vi "Array Max & Min PtByPt.vi"(0 "input data point":dbl format="%0.2f", 1 "sample length":i32=100, 2 "initialize":bool) -> (3 "error":i32, 4 "max index":i32, 5 "max value":dbl format="%0.2f", 6 "min index":i32, 7 "min value":dbl format="%0.2f")   [LabVIEW 2020, in "NI_PtbyPt.lvlib"]
doc: "Searches for the maximum and minimum values in the set of input data points specified by <B>sample length</B> where the region of interest is determined by the last <B>sample length</B> data. The indexes are between 0 and <B>sample length</B>."
uses:
  NI_PtbyPt.lvlib
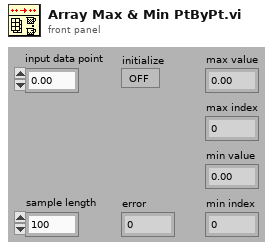
[diagram p1: front panel]
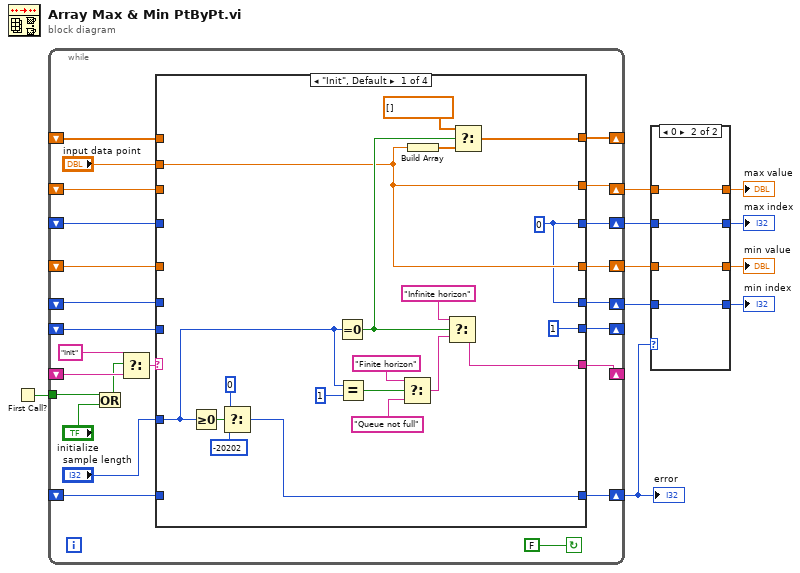
[diagram p0: block diagram]
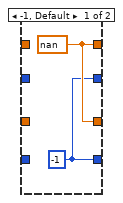
[diagram p2: hidden frame]
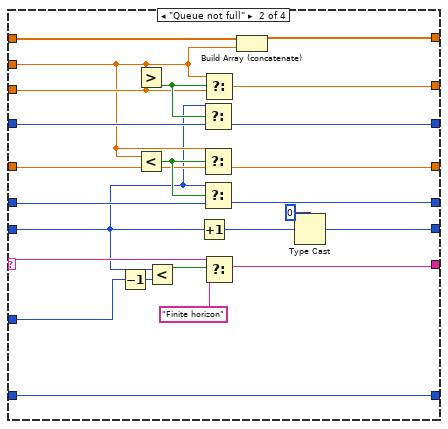
[diagram p3: hidden frame]
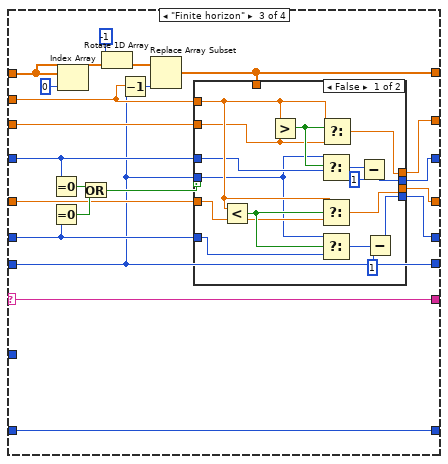
[diagram p4: hidden frame]
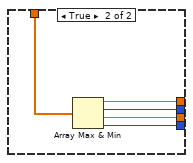
[diagram p5: hidden frame]
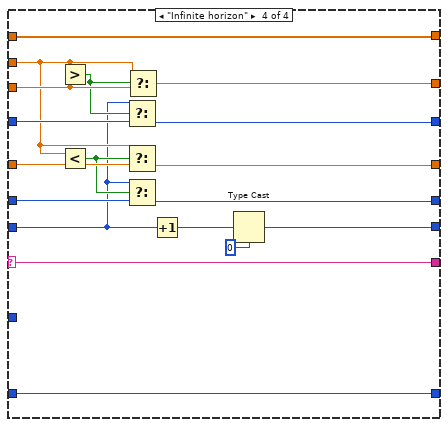
[diagram p6: hidden frame]
diagram:
  n1 = First Call?() -> (First Call?: T/F=w10:bool)
  n2 = while {
    tunnel: w10 -> [w15]
    shift-left: _ -> [w19]
    shift-right: [w22] -> w6
    shift-left: _ -> [w20]
    shift-right: [w21] -> w4
    shift-left: _ -> [w24]
    shift-right: [w23] -> w2
    shift-left: _ -> [w26]
    shift-right: [w25] -> _
    shift-left: _ -> [w28]
    shift-right: [w29] -> _
    shift-left: _ -> [w30]
    shift-right: [w31] -> w9
    shift-left: _ -> [w34]
    shift-right: [w27] -> _
    shift-right: [w12] -> w7
    shift-left: _ -> [w11]
    stop <- FALSE continue-if-true
    n3 = Or(x=w15, y="initialize") -> (x .or. y?=w13:bool)
    n4 = Select(t="Init", s=w13, f=w34) -> (s? t:f=w32:string)
    n5 = case shown="\"Init\", Default" w32 {
      selector: w32 -> [_ w70 w94 w137]
      tunnel: [w40 w60 w80 w125] -> w31
      tunnel: w30 -> [_ w61 w82 w126]
      tunnel: "input data point" -> [w41 w56 w86 w130]
      tunnel: [1 w74 w81 w122] -> w29
      tunnel: w28 -> [_ w55 w81 w124]
      tunnel: [w46 w68 w94 w137] -> w27
      tunnel: w26 -> [_ w77 w88 w136]
      tunnel: [w42 w76 w87 w136] -> w25
      tunnel: "sample length" -> [w38 w72 _ _]
      tunnel: w24 -> [_ w64 w85 w135]
      tunnel: [w41 w57 w90 w134] -> w23
      tunnel: [w41 w59 w89 w128] -> w22
      tunnel: [w40 w58 w79 w131] -> w21
      tunnel: w20 -> [_ w63 w84 w133]
      tunnel: w19 -> [_ w62 w83 w129]
      tunnel: [w35 w54 w78 w120] -> w12
      tunnel: w11 -> [_ w54 w78 w120]
      frame "Init", Default {
        w40 = 0
        n6 = Greater Or Equal To 0?(x=w38) -> (x >= 0?=w39:bool)
        n7 = Select(t=0, s=w39, f=-20202) -> (s? t:f=w35:i32)
        n8 = Equal To 0?(x=w38) -> (x = 0?=w45:bool)
        n9 = Equal?(x=w38, y=1) -> (x = y?=w50:bool)
        n10 = Select(t="Finite horizon", s=w50, f="Queue not full") -> (s? t:f=w48:string)
        n11 = Build Array(w41) -> (w44:dbl[])
        n12 = Select(t="Infinite horizon", s=w45, f=w48) -> (s? t:f=w46:string)
        n13 = Select(t=dbl[] [], s=w45, f=w44) -> (s? t:f=w42:dbl[])
      }
      frame "Queue not full" {
        n14 = Decrement(x=w72) -> (x-1=w67:i32)
        n15 = Greater?(x=w56, y=w64) -> (0:w66:bool)
        n16 = Less?(x=w56, y=w62) -> (x < y?=w65:bool)
        n17 = Less?(x=w55, y=w67) -> (x < y?=w71:bool)
        n18 = Increment(x=w55) -> (x+1=w75:i32)
        n19 = Select(t=w55, s=w66, f=w63) -> (s? t:f=w58:i32)
        n20 = Select(t=w56, s=w65, f=w62) -> (s? t:f=w59:dbl)
        n21 = Select(t=w55, s=w65, f=w61) -> (s? t:f=w60:i32)
        n22 = Select(t=w56, s=w66, f=w64) -> (s? t:f=w57:dbl)
        n23 = Select(t=w70, s=w71, f="Finite horizon") -> (s? t:f=w68:string)
        n24 = Build Array (concatenate)(w77, w56) -> (w76:dbl[])
        n25 = Type Cast(type=0, x=w75) -> (*(type *) &x=w74:i32)
      }
      frame "Finite horizon" {
        n26 = Equal To 0?(x=w84) -> (x = 0?=w93:bool)
        n27 = Equal To 0?(x=w82) -> (x = 0?=w92:bool)
        n28 = Index Array(array=w88, index=0 ("Index")) -> ()  [unwired: 1 out]
        n29 = Or(x=w93, y=w92) -> (x .or. y?=w91:bool)
        n30 = Rotate 1D Array(1:w88, 2:i16 -1 ("n")) -> (0:w96:dbl[])
        n31 = Decrement(x=w81) -> (x-1=w95:i32)
        n32 = Replace Array Subset(array=w96, new element=w86, index=w95) -> (w87:dbl[])
        n33 = case shown="False" w91 {
          tunnel: w87 -> [_ w119]
          tunnel: [w107 w118] -> w90
          tunnel: [w103 w117] -> w79
          tunnel: [w106 w116] -> w89
          tunnel: [w99 w115] -> w80
          tunnel: w86 -> [w112 _]
          tunnel: w85 -> [w111 _]
          tunnel: w84 -> [w108 _]
          tunnel: w83 -> [w110 _]
          tunnel: w82 -> [w109 _]
          tunnel: w81 -> [w105 _]
          frame False {
            n34 = Less?(x=w112, y=w110) -> (x < y?=w113:bool)
            n35 = Greater?(x=w112, y=w111) -> (0:w114:bool)
            n36 = Select(t=w105, s=w114, f=w108) -> (s? t:f=w104:i32)
            n37 = Select(t=w112, s=w113, f=w110) -> (s? t:f=w106:dbl)
            n38 = Select(t=w105, s=w113, f=w109) -> (s? t:f=w101:i32)
            n39 = Select(t=w112, s=w114, f=w111) -> (s? t:f=w107:dbl)
            n40 = Subtract(x=w104, y=1) -> (x-y=w103:i32)
            n41 = Subtract(x=w101, y=1) -> (x-y=w99:i32)
          }
          frame True {
            n42 = Array Max & Min(array=w119) -> (max value=w118:dbl, max index (indices)=w117:i32, min value=w116:dbl, min index (indices)=w115:i32)
          }
        }
      }
      frame "Infinite horizon" {
        n43 = Greater?(x=w130, y=w135) -> (0:w132:bool)
        n44 = Less?(x=w130, y=w129) -> (x < y?=w127:bool)
        n45 = Select(t=w124, s=w132, f=w133) -> (s? t:f=w131:i32)
        n46 = Select(t=w130, s=w127, f=w129) -> (s? t:f=w128:dbl)
        n47 = Select(t=w124, s=w127, f=w126) -> (s? t:f=w125:i32)
        n48 = Select(t=w130, s=w132, f=w135) -> (s? t:f=w134:dbl)
        n49 = Increment(x=w124) -> (x+1=w123:i32)
        n50 = Type Cast(type=0, x=w123) -> (*(type *) &x=w122:i32)
      }
    }
  }
  "error" <- w7
  n51 = case shown="0" w7 {
    tunnel: w9 -> [_ w143]
    tunnel: [w138 w143] -> w8
    tunnel: w6 -> [_ w142]
    tunnel: [w139 w142] -> w5
    tunnel: w4 -> [_ w141]
    tunnel: [w138 w141] -> w3
    tunnel: w2 -> [_ w140]
    tunnel: [w139 w140] -> w1
    frame -1, Default {
      w138 = -1
      w139 = nan ("input data point")
    }
    frame 0 {
    }
  }
  "max index" <- w3
  "min index" <- w8
  "max value" <- w1
  "min value" <- w5
